vi "OptimizePointSetFromPointSetCorrespondenceTransforms.vi"(7 "Point Set Weights":dbl[](array[numeric]), 8 "error in (no error)":errorcluster, 9 "Sum (v * C^2)":dbl, 10 "Transforms":T1[](array[typedef]), 11 "Point Corespondences":dbl[][][](array[numeric])) -> (0 "error out":errorcluster, 2 "LMS Error":dbl, 3 "Optimized Points":dbl[][](array[numeric]))   [LabVIEW 2020, in "ar.lvlib"]
uses:
  ar.lvlib
  Transform.ctl
  <vilib>/Analysis/Matrix/Datatypes/RealMatrix.ctl
  <vilib>/Analysis/baseanly.llb/A x Vector.vi
  <vilib>/Analysis/NI_AALBase.lvlib
  <vilib>/Analysis/Matrix/NI_Matrix.lvlib
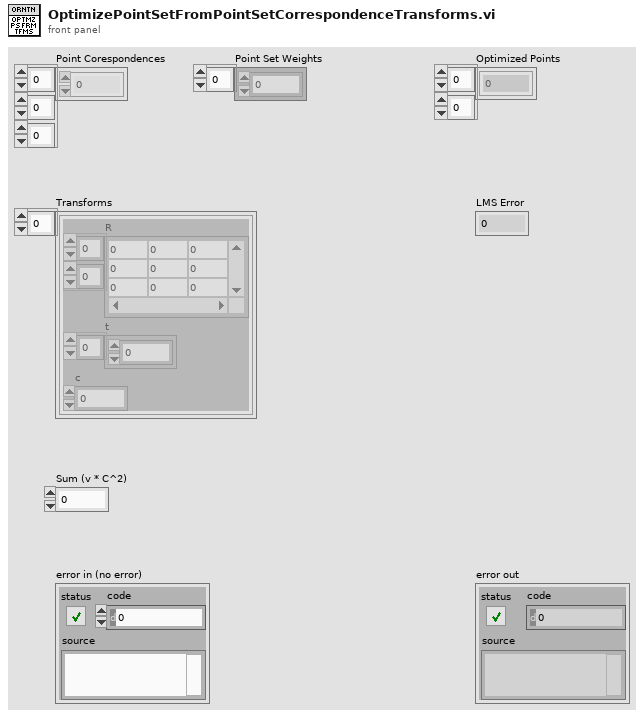
[diagram p1: front panel]
types:
  T1 = typedef "ar.lvlib/Transform.ctl" = cluster{"R":T2, "t":dbl[], "c":dbl}
  T2 = typedef "NI_Matrix.lvlib/RealMatrix.ctl" = dbl[][]
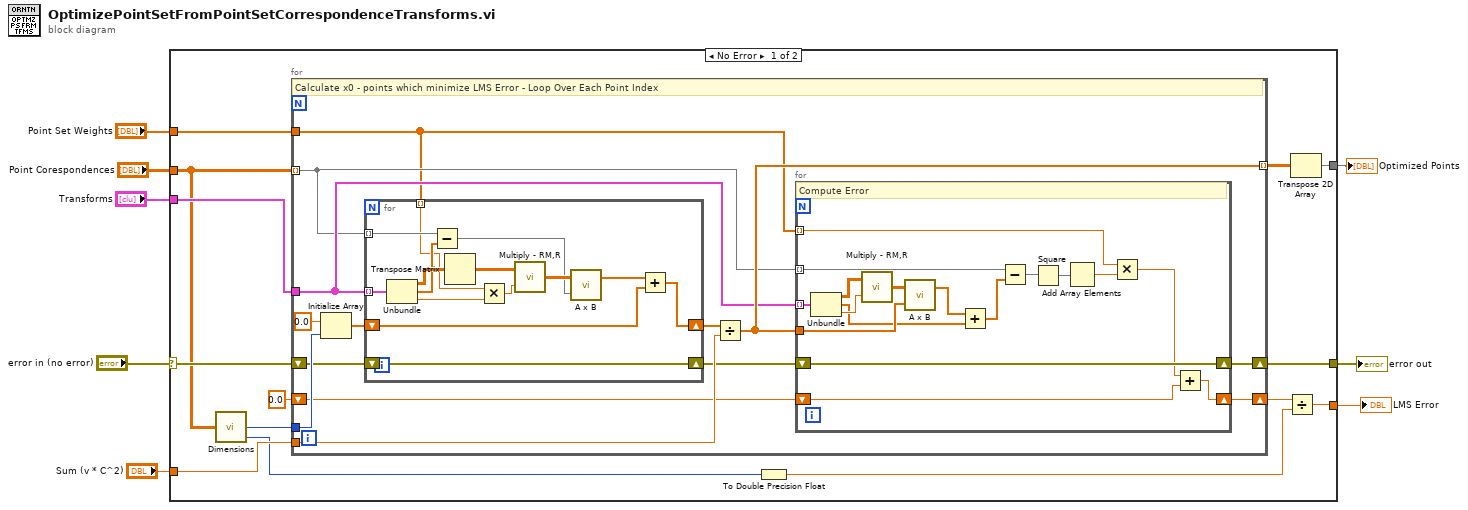
[diagram p0: block diagram]
diagram:
  n1 = case shown="No Error" "error in (no error)" {
    selector: "error in (no error)" -> [w16 _]
    tunnel: "Sum (v * C^2)" -> [w22 _]
    tunnel: "Point Corespondences" -> [w14 _]
    tunnel: "Transforms" -> [w19 _]
    tunnel: [w18 _] -> w5
    tunnel: [w11 _] -> w4
    tunnel: [w17 _] -> w3
    tunnel: "Point Set Weights" -> [w15 _]
    frame No Error {
      n2 = call "Dimensions.vi"("Corresponding Object Points Array"=w14) -> ("m dimensions"=w13:i32, "n points in a point set"=w10:i32)  [unwired: 1 in, 1 out]
      n3 = for {
        tunnel: w14 -> [w29] mode=indexing
        tunnel: w19 -> [w30]
        tunnel: w22 -> [w32]
        tunnel: w13 -> [w36]
        tunnel: [w31] -> w20 mode=indexing
        shift-right: [w27] -> w12
        shift-left: 0.0 -> [w28]
        shift-right: [w24] -> w17
        shift-left: w16 -> [w26]
        tunnel: w15 -> [w23]
        # "Calculate x0 - points which minimize LMS Error - Loop Over Each Point Index"
        n4 = Initialize Array(0.0 ("element"), w36) -> (w34:dbl[])
        n5 = for {
          tunnel: w29 -> [w63] mode=indexing
          tunnel: w30 -> [w67] mode=indexing
          shift-right: [w57] -> w33
          shift-left: w34 -> [w58]
          shift-right: [w56] -> w25
          shift-left: w26 -> [w56]
          tunnel: w23 -> [w54] mode=indexing
          n6 = Unbundle(w67) -> ("R"=w66:T2, "t"=w62:dbl[], "c"=w64:dbl)
          n7 = Subtract(x=w63, y=w62) -> (x-y=w60:dbl[])
          n8 = Transpose Matrix(1:w66) -> (0:w65:T2)
          n9 = Multiply(x=w54, y=w64) -> (x*y=w55:dbl)
          n10 = call <vilib>:"Multiply - RM,R.vi"("Real Scalar c"=w55, "Real Matrix A"=w65) -> ("A * c"=w61:T2)
          n11 = call-poly <vilib>:"A x B.vi"("Vector"=w60, "A"=w61) -> ("A x Vector"=w59:dbl[])  [unwired: 1 out]
          n12 = Add(x=w59, y=w58) -> (x+y=w57:dbl[])
        }
        n13 = Divide(x=w33, y=w32) -> (x/y=w31:dbl[])
        n14 = for {
          tunnel: w31 -> [w49]
          tunnel: w30 -> [w53] mode=indexing
          tunnel: w29 -> [w46] mode=indexing
          shift-right: [w41] -> w27
          shift-left: w28 -> [w42]
          shift-right: [w40] -> w24
          shift-left: w25 -> [w40]
          tunnel: w23 -> [w38] mode=indexing
          # "Compute Error"
          n15 = Unbundle(w53) -> ("R"=w52:T2, "t"=w47:dbl[], "c"=w51:dbl)
          n16 = call <vilib>:"Multiply - RM,R.vi"("Real Scalar c"=w51, "Real Matrix A"=w52) -> ("A * c"=w50:T2)
          n17 = call-poly <vilib>:"A x B.vi"("Vector"=w49, "A"=w50) -> ("A x Vector"=w48:dbl[])  [unwired: 1 out]
          n18 = Add(x=w48, y=w47) -> (x+y=w45:dbl[])
          n19 = Subtract(x=w46, y=w45) -> (x-y=w44:dbl[])
          n20 = Square(x=w44) -> (x^2=w43:dbl[])
          n21 = Add Array Elements(numeric array=w43) -> (sum=w37:dbl)
          n22 = Multiply(x=w38, y=w37) -> (x*y=w39:dbl)
          n23 = Add(x=w39, y=w42) -> (x+y=w41:dbl)
        }
      }
      n24 = To Double Precision Float(number=w10) -> (double precision float=w9:dbl)
      n25 = Divide(x=w12, y=w9) -> (x/y=w11:dbl)
      n26 = Transpose 2D Array(2D array=w20) -> (transposed array=w18:dbl[][])
    }
    frame Error {
    }
  }
  "Optimized Points" <- w5
  "LMS Error" <- w4
  "error out" <- w3
